vi "Photometer linear fit.vi"(10 "Photometer data in":T1, 11 "Absorbance":dbl) -> (0 "XY Graph":cluster{"Best Linear Fit":dbl[], dbl[]}[](graph), 1 "R-square":dbl, 2 "intercept":dbl, 3 "slope":dbl)   [LabVIEW 2015]
uses:
  Photometer calibration data.ctl
  <vilib>/Analysis/NI_AALPro.lvlib
panel:
  out "Concentration":dbl
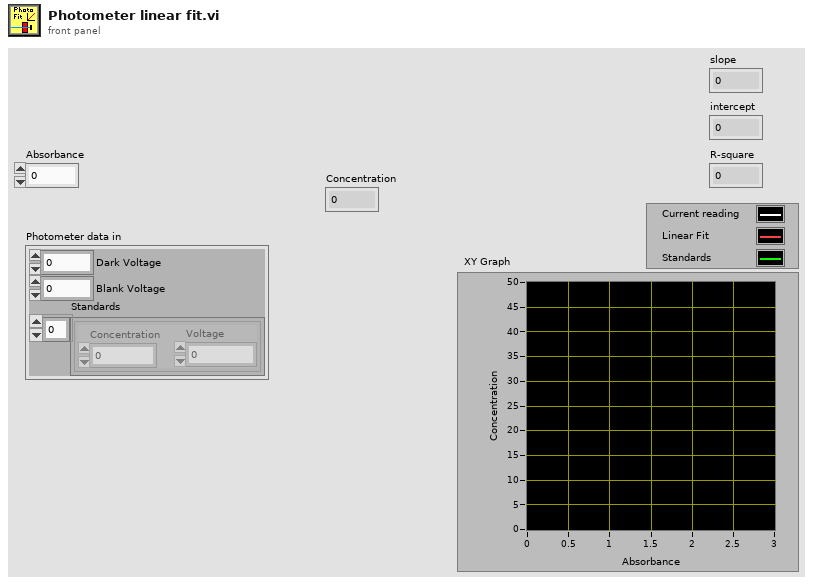
[diagram p1: front panel]
types:
  T1 = typedef "Photometer calibration data.ctl" = cluster{"Dark Voltage":dbl, "Blank Voltage":dbl, "Standards":cluster{"Concentration":dbl, "Voltage":dbl}[]}
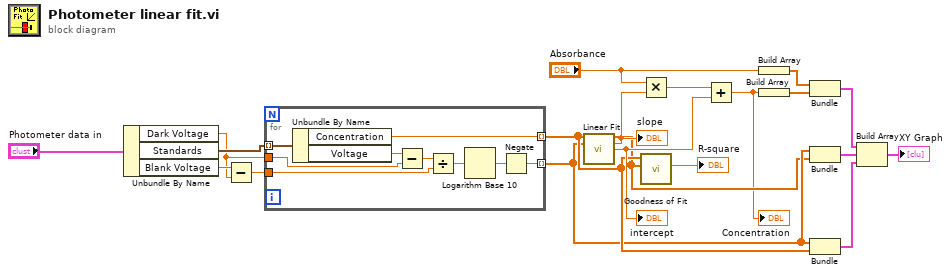
[diagram p0: block diagram]
diagram:
  n1 = Unbundle By Name("Photometer data in") -> ("Dark Voltage"=w17:dbl, "Standards"=w19:cluster{"Concentration":dbl, "Voltage":dbl}[], "Blank Voltage"=w18:dbl)
  n2 = Subtract(x=w18, y=w17) -> (x-y=w8:dbl)
  n3 = for {
    tunnel: w19 -> [w29] mode=indexing
    tunnel: w17 -> [w27]
    tunnel: w8 -> [w23]
    tunnel: [w22] -> w6 mode=indexing
    tunnel: [w21] -> w7 mode=indexing
    n4 = Unbundle By Name(w29) -> ("Concentration"=w21:dbl, "Voltage"=w28:dbl)
    n5 = Subtract(x=w28, y=w27) -> (x-y=w26:dbl)
    n6 = Divide(x=w26, y=w23) -> (x/y=w25:dbl)
    n7 = Logarithm Base 10(1:w25) -> (0:w24:dbl)
    n8 = Negate(x=w24) -> (-x=w22:dbl)
  }
  n9 = call <vilib>:"Linear Fit.vi"("Y"=w7, "X"=w6) -> ("Best Linear Fit"=w5:dbl[], "slope"=w15:dbl, "intercept"=w14:dbl)  [unwired: 9 in, 2 out]
  "intercept" <- w14
  "slope" <- w15
  n10 = Multiply(x="Absorbance", y=w15) -> (x*y=w16:dbl)
  n11 = call <vilib>:"Goodness of Fit.vi"("Best Fit"=w5, "Y"=w7) -> ("R-square"=→"R-square":dbl)  [unwired: 6 in, 3 out]
  n12 = Add(x=w16, y=w14) -> (x+y=w4:dbl)
  "Concentration" <- w4
  n13 = Build Array("Absorbance") -> (w12:dbl[])
  n14 = Build Array(w4) -> (w10:dbl[])
  n15 = Bundle(w12, w10) -> (w11:cluster{dbl[], dbl[]})  [unwired: 1 in]
  n16 = Bundle(w6, "Best Linear Fit"=w5) -> (w2:cluster{dbl[], "Best Linear Fit":dbl[]})  [unwired: 1 in]
  n17 = Bundle(w6, w7) -> (w1:cluster{dbl[], dbl[]})  [unwired: 1 in]
  n18 = Build Array(w11, w2, w1) -> (→"XY Graph":cluster{dbl[], "Best Linear Fit":dbl[]}[])
